vi "(SubVI)Waveform Editor_Export Manager.vi"(7 "Enable Memory":bool, 8 "error in (no error)":errorcluster caption="에러 입력(에러 없음)", 10 "Sampling Rate":u32 caption="Sampling Rate :", 11 "WF List":T1[](array[typedef])) -> (0 "error out":errorcluster caption="에러 출력")   [LabVIEW 2020]
uses:
  Controls/(Ctrl)Waveform Editor_WF List.ctl
  Libraries/Waveform Obj Class/Waveform Obj/Waveform Obj.lvclass
  <vilib>/Utility/miscctls.llb/LVPointTypeDef.ctl
  Control Data/Controls/(Ctrl)Control Data_Save or Load Control Data_Function.ctl
  <vilib>/Utility/miscctls.llb/LVStringsAndValuesArrayTypeDef_I32.ctl
  Libraries/Haptic IC Class/Haptic IC/Haptic IC.lvclass/Haptic IC.ctl
  Variables/(Var)System Variables.vi
  Libraries/Haptic IC Class/Haptic IC/Haptic IC.lvclass
panel:
  in  "Export":bool
  in  "File Format":enum32{"TXT", "WAV"}(tab)
  out "Text_Sampling Rate":u32 caption="Sampling Rate" format="%#pHz"
  in  "TXT_EOL+Delimiter":bool=TRUE
  in  "TXT_Number per Line":i32=1 caption="Number per Line" min=1 max=100
  in  "TXT_End of LIne":enum16{"EOL (\\r\\n)", "LF (\\n)"}(ring) caption="End of Line"
  in  "TXT_Delimiter":string(combo)="\r\n" caption="Delimiter"
  in  "TXT_Prefix":bool=TRUE
  in  "TXT_Waveform No.":i32(ring) caption="Waveform No."
  in  "TXT_Radix":enum16{"BIN", "DEC", "HEX"}(ring)=enum."HEX" caption="Radix"
  out "TXT_Preview":string caption="Preview"
  in  "WAV_Preview Data Type":enum16{"±1", "8bit"}(ring) caption="Preview"
  in  "WAV_Waveform No.":i32(ring) caption="Waveform No."
  out "WAV_Sampling Rate":u32 caption="Sampling Rate" format="%#pHz"
  out "WAV_Bits Per Sample":i32(ring)=8 caption="Bits / Sample" items=["8"=8, "16"=16, "24"=24, "32"=32]
  out "WAV_Preview":waveform(dbl)(graph) caption="Preview"
  # "Export Manager"
  # "Sound Format"
  # "Data Format"
  # "Preview"
  # "Data"
  # "Data Format"
  # "Data"
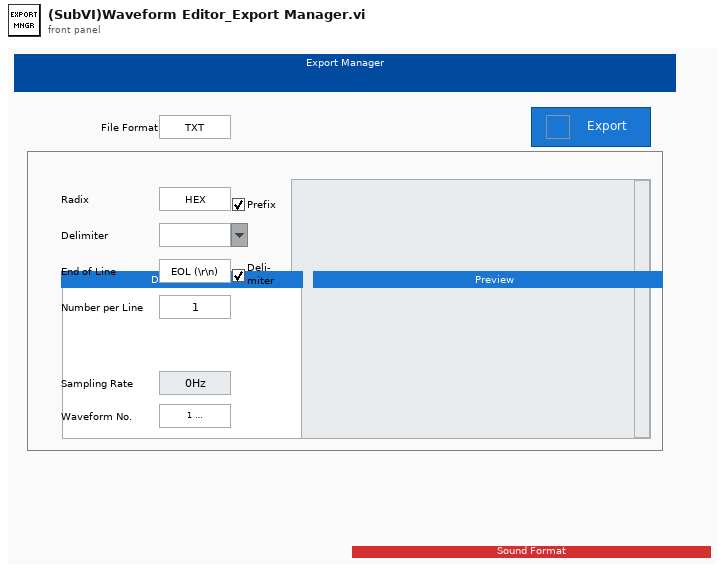
[diagram p1: front panel]
types:
  T1 = typedef "(Ctrl)Waveform Editor_WF List.ctl" = cluster{"Name":string, "WF Seq":refnum<class "Waveform Obj.lvclass">[]}
  T2 = typedef "LVPointTypeDef.ctl" = cluster{"Horizontal":i16, "Vertical":i16}
  T3 = typedef "(Ctrl)Control Data_Save or Load Control Data_Function.ctl" = enum16{"Save", "Load"}
  T4 = typedef "LVStringsAndValuesArrayTypeDef_I32.ctl" = cluster{"String":string, "Value":i32}[]
  T5 = typedef "Haptic IC.lvclass/(Ctrl)IC Type.ctl" = enum8{"DW7800", "DW7802", "DW7912", "DW7914"}
  T6 = enum8{"Enabled", "Disabled", "Disabled and Grayed Out"}
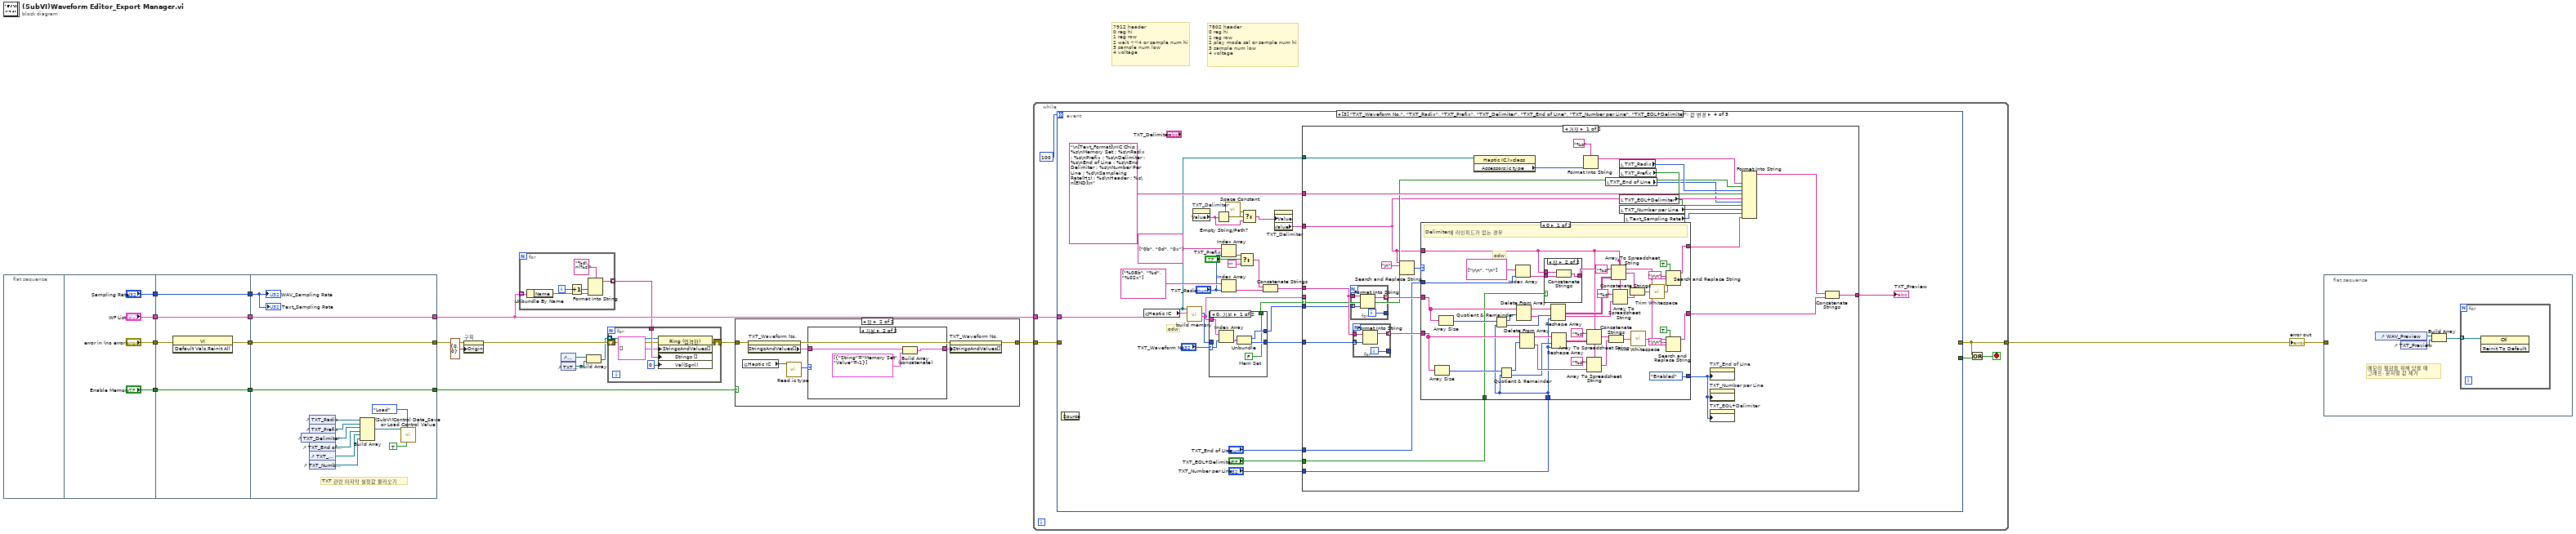
[diagram p0: block diagram]
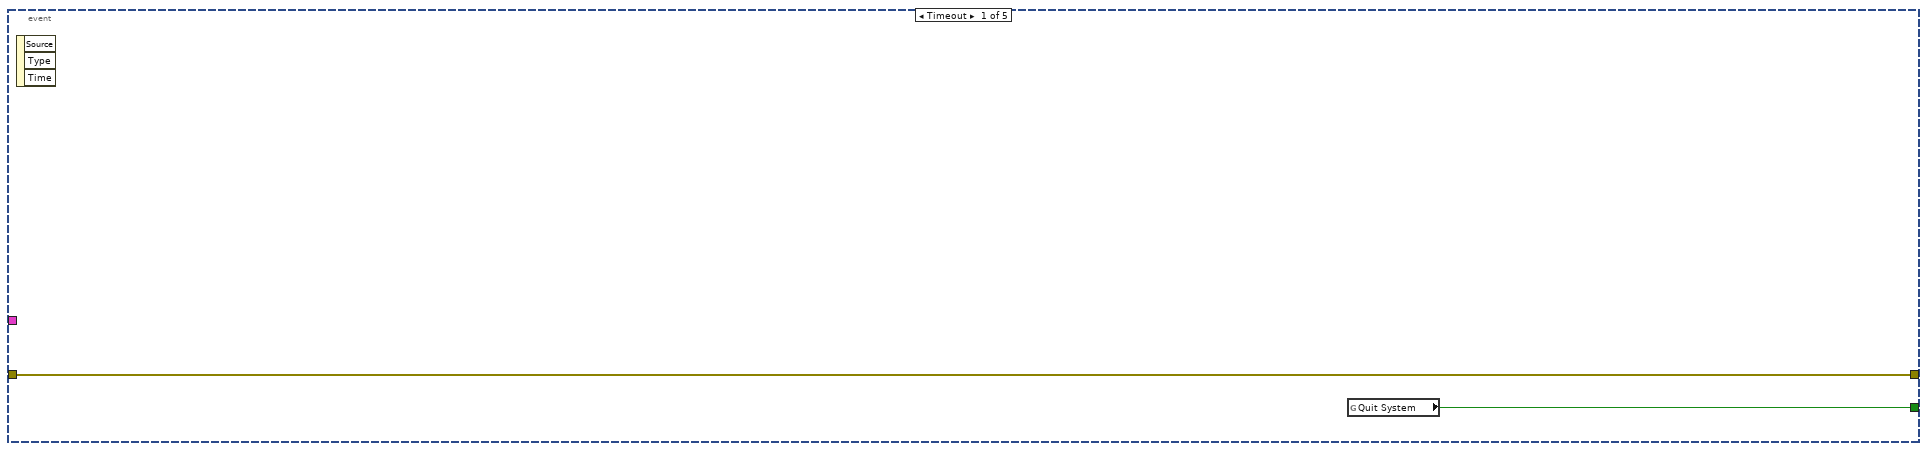
[diagram p4: hidden frame]
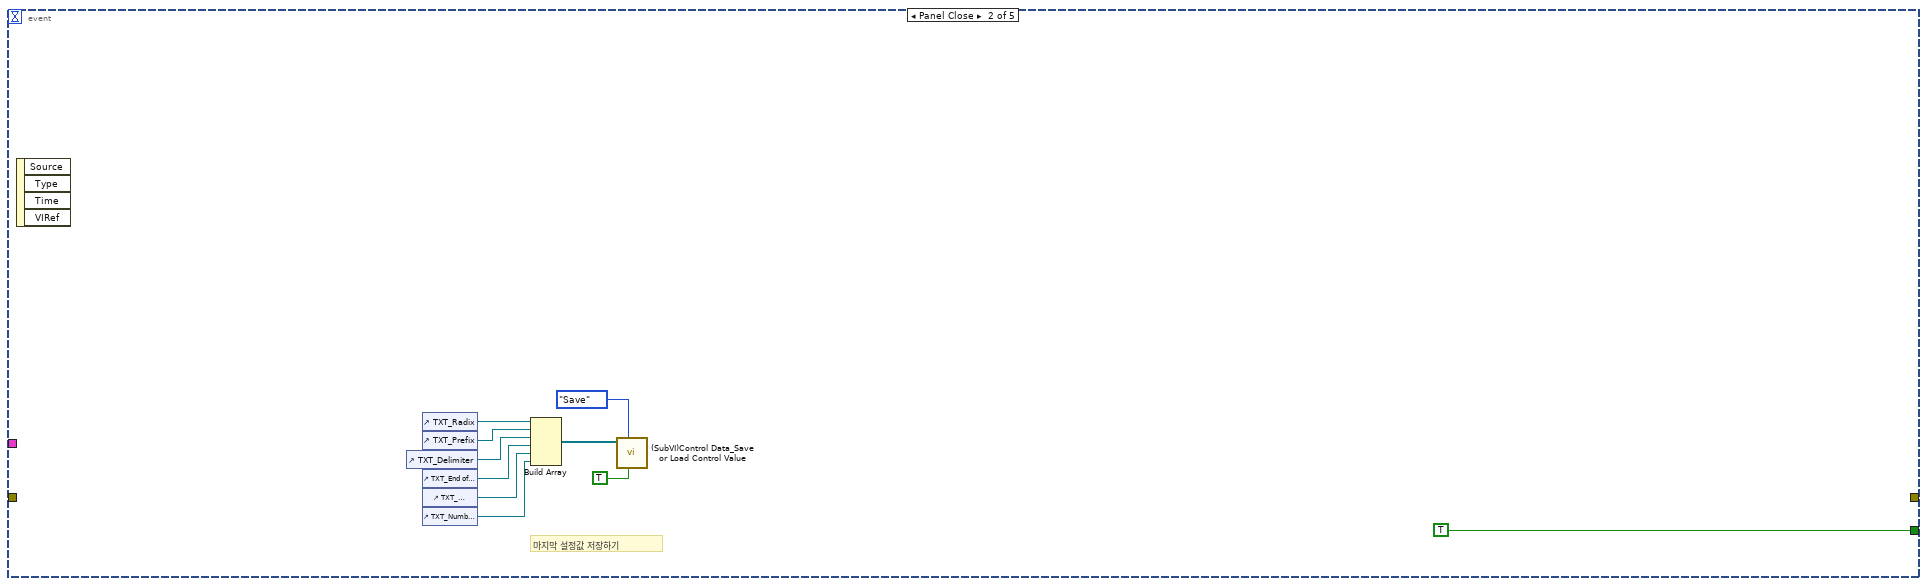
[diagram p5: hidden frame]
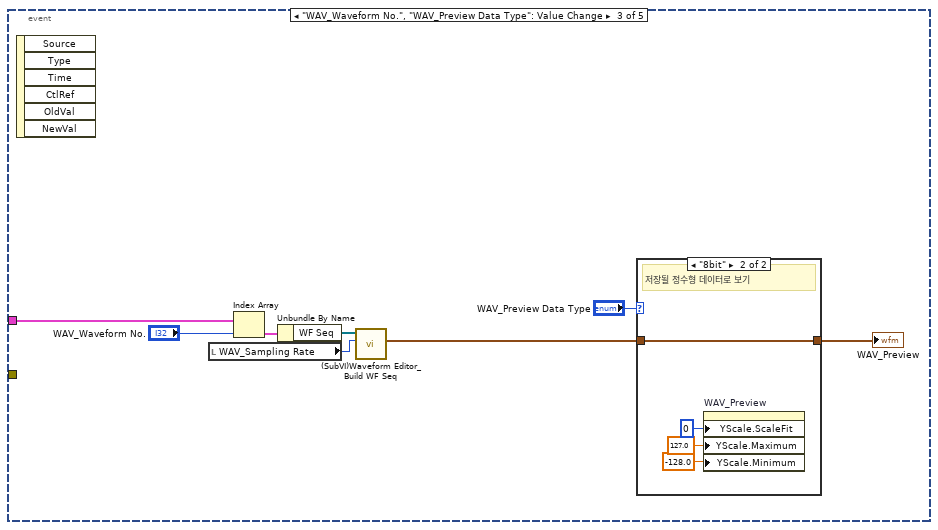
[diagram p6: hidden frame]
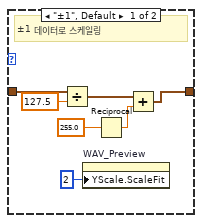
[diagram p7: hidden frame]
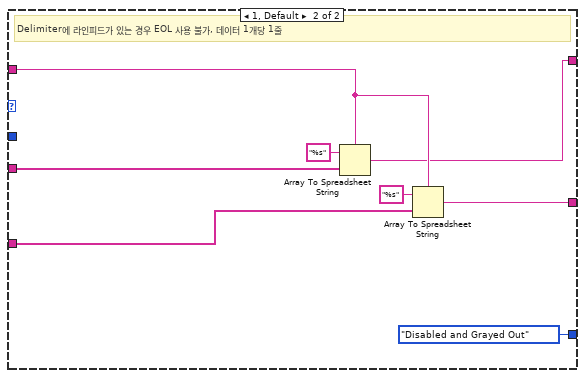
[diagram p9: hidden frame]
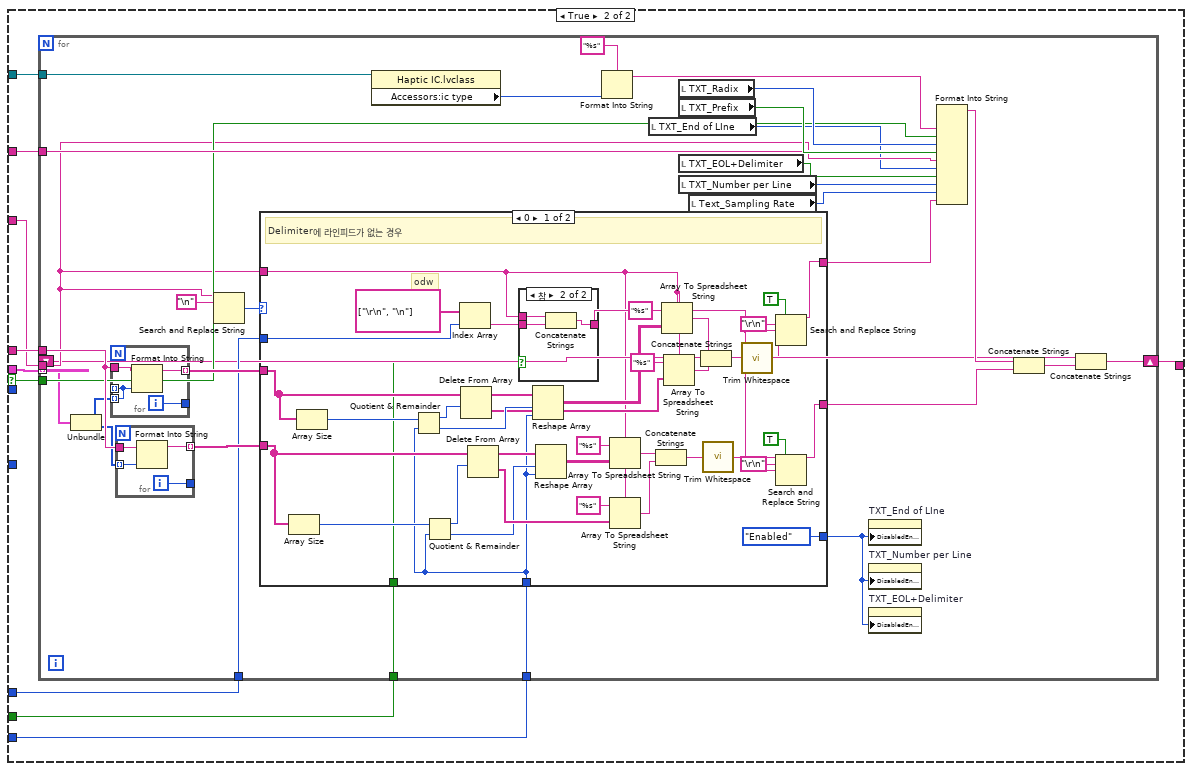
[diagram p10: hidden frame]
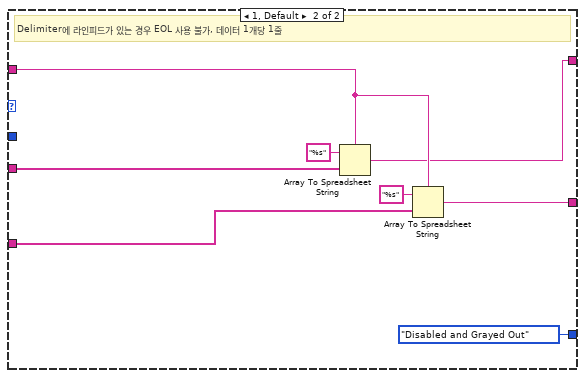
[diagram p12: hidden frame]
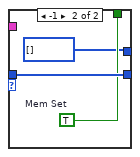
[diagram p13: hidden frame]
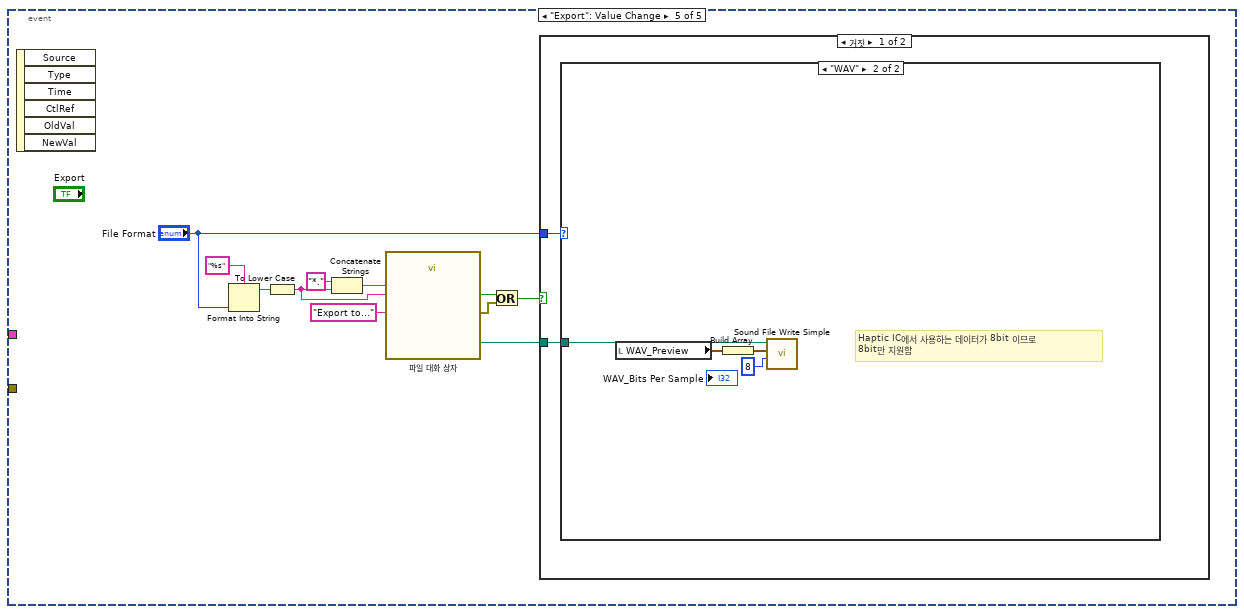
[diagram p14: hidden frame]
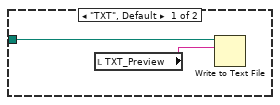
[diagram p15: hidden frame]
diagram:
  # "7802 header\n0 reg hi\n1 reg row\n2 play mode cal or sample num hi\n3 sample num low\n4 voltage"
  # "7912 header\n0 reg hi\n1 reg row\n2 wait <<4 or sample num hi\n3 sample num low\n4 voltage"
  n1 = flat-sequence {
    tunnel: ["error in (no error)"] -> w16
    tunnel: ["WF List"] -> w15
    tunnel: ["Sampling Rate"] -> w10
    tunnel: ["Enable Memory"] -> w1
    tunnel: w16 -> [w28]
    tunnel: w15 -> [w29]
    tunnel: [w29] -> w13
    tunnel: [w27] -> w12
    tunnel: [w26] -> w11
    tunnel: w10 -> [w26]
    tunnel: [w25] -> w2
    tunnel: w1 -> [w25]
    tunnel: [w41] -> w14
    tunnel: [w42] -> w19
    tunnel: w13 -> [w42]
    tunnel: w12 -> [w41]
    tunnel: w11 -> [w30]
    tunnel: [w31] -> w3
    tunnel: w2 -> [w31]
    frame #0 {
    }
    frame #1 {
    }
    frame #2 {
      n2 = invoke class="VI" method="Default Vals.Reinit All"(error in=w28) -> (error out=w27:errorcluster)  [unwired: 2 in, 2 out]
    }
    frame #3 {
      # "TXT 관련 마지막 설정값 불러오기"
      n3 = control-ref of="TXT_Delimiter"() -> (w37:refnum<vi>)
      n4 = control-ref of="TXT_Radix"() -> (w35:refnum<vi>)
      n5 = control-ref of="TXT_Prefix"() -> (w36:refnum<vi>)
      n6 = control-ref of="TXT_End of LIne"() -> (w38:refnum<vi>)
      n7 = control-ref of="TXT_EOL+Delimiter"() -> (w39:refnum<vi>)
      n8 = control-ref of="TXT_Number per Line"() -> (w40:refnum<vi>)
      n9 = Build Array(w35, w36, w37, w38, w39, w40) -> (w33:refnum<vi>[])
      n10 = call "(SubVI)Control Data_Save or Load Control Value.vi"("Common? (f)"=TRUE, "Function"=(Ctrl)Control_Data_Save_or_Load_Control_Data_Function."Load", "Control Ref"=w33) -> ()  [unwired: 8 in, 1 out]
      "WAV_Sampling Rate" <- w30
      "Text_Sampling Rate" <- w30
    }
  }
  n11 = property on="구획" class="Pane"(error in=w14, "Origin"=T2 {"Horizontal"=0, "Vertical"=0} ("원점")) -> (error out=w17:errorcluster)  [unwired: 1 in, 1 out]
  n12 = for {
    tunnel: w19 -> [w48] mode=indexing
    tunnel: [w44] -> w18 mode=indexing
    i -> [w46]
    n13 = Unbundle By Name(w48) -> ("Name"=w47:string)
    n14 = Increment(x=w46) -> (x+1=w43:i32)
    n15 = Format Into String(format string="%d\n(%s)" ("포맷 문자열"), w43, w47) -> (resulting string=w44:string)  [unwired: 2 in, 1 out]
  }
  n16 = control-ref of="WAV_Waveform No."() -> (w9:refnum<vi>)
  n17 = control-ref of="TXT_Waveform No."() -> (w8:refnum<vi>)
  n18 = Build Array(w9, w8) -> (w7:refnum<vi>[])
  n19 = for {
    tunnel: w18 -> [w54]
    tunnel: w7 -> [w50] mode=indexing
    shift-right: [w52] -> w5
    shift-left: w17 -> [w53]
    n20 = property on="프로퍼티 노드" class="Ring (엄격한)"(reference=w50, error in=w53, "StringsAndValues[]"=T4 [] ("문자열과 값[]"), "Strings []"=w54, "Val(Sgnl)"=0 ("값(신호)")) -> (error out=w52:errorcluster)  [unwired: 1 out]
  }
  n21 = case shown="참" w3 {
    tunnel: w5 -> [w55 w62]
    tunnel: [w55 w60] -> w4
    frame False {
    }
    frame True {
      n22 = global read "(Var)System Variables.vi" "Haptic IC"() -> (w57:refnum<class "Haptic IC.lvclass">)
      n23 = property on="TXT_Waveform No." class="Ring (엄격한)"(error in=w62) -> (error out=w61:errorcluster, "StringsAndValues[]"=w59:T4)  [unwired: 1 in, 1 out]
      n24 = call "Read ic type.vi"("Haptic IC 입력"=w57) -> ("ic type"=w56:T5)  [unwired: 8 in, 2 out]
      n25 = case shown="기본" w56 {
        tunnel: w59 -> [w63 w66]
        tunnel: [w63 w64] -> w58
        frame "DW7800" {
          # "Memory를 사용하지 않는 IC의 경우 (DW7800)\nMemory Set 없이 개별 Waveform 데이터만 사용"
        }
        frame Default {
          n26 = Build Array (concatenate)(w66, T4 [{"String"="Memory Set", "Value"=-1}] ("배열")) -> (w64:T4)
        }
      }
      n27 = property on="TXT_Waveform No." class="Ring (엄격한)"(error in=w61, "StringsAndValues[]"=w58) -> (error out=w60:errorcluster)  [unwired: 1 in, 1 out]
    }
  }
  n28 = while {
    tunnel: w4 -> [w71]
    tunnel: [w70] -> w6
    tunnel: w19 -> [w67]
    stop <- w69 stop-if-true
    n29 = event shown="[3] \"TXT_Waveform No.\", \"TXT_Radix\", \"TXT_Prefix\", \"TXT_Delimiter\", \"TXT_End of LIne\", \"TXT_Number per Line\", \"TXT_EOL+Delimiter\": 값 변경" {
      selector: _ -> [_ _ _ _ _]
      dyn-events: _ -> [_ _ _ _ _]
      timeout: 100 -> [_ _ _ _ _]
      tunnel: [w74 _ _ _ _] -> w70
      tunnel: w71 -> [w74 _ _ _ _]
      tunnel: [w73 TRUE _ _ _] -> w68
      tunnel: w67 -> [_ _ w92 w115 _]
      event Timeout {
        n30 = event-data() -> ()  [unwired: 1 in, 3 out]
        n31 = global read "(Var)System Variables.vi" "Quit System"() -> (w73:bool)
      }
      event Panel Close {
        # "마지막 설정값 저장하기"
        n32 = event-data() -> ()  [unwired: 1 in, 4 out]
        n33 = control-ref of="TXT_Delimiter"() -> (w78:refnum<vi>)
        n34 = control-ref of="TXT_Radix"() -> (w80:refnum<vi>)
        n35 = control-ref of="TXT_Prefix"() -> (w79:refnum<vi>)
        n36 = control-ref of="TXT_End of LIne"() -> (w77:refnum<vi>)
        n37 = control-ref of="TXT_EOL+Delimiter"() -> (w76:refnum<vi>)
        n38 = control-ref of="TXT_Number per Line"() -> (w75:refnum<vi>)
        n39 = Build Array(w80, w79, w78, w77, w76, w75) -> (w82:refnum<vi>[])
        n40 = call "(SubVI)Control Data_Save or Load Control Value.vi"("Common? (f)"=TRUE, "Function"=(Ctrl)Control_Data_Save_or_Load_Control_Data_Function."Save", "Control Ref"=w82) -> ()  [unwired: 8 in, 1 out]
      }
      event "WAV_Waveform No.", "WAV_Preview Data Type": Value Change {
        n41 = event-data() -> ()  [unwired: 1 in, 6 out]
        n42 = local read "WAV_Sampling Rate"() -> (w87:u32)
        n43 = Index Array(array=w92, index="WAV_Waveform No.") -> (element=w90:T1)
        n44 = Unbundle By Name(w90) -> ("WF Seq"=w89:refnum<class "Waveform Obj.lvclass">[])
        n45 = call "(SubVI)Waveform Editor_Build WF Seq.vi"("Sampling Rate"=w87, "WF Seq"=w89) -> ("waveform out"=w86:waveform(i8))  [unwired: 4 in, 5 out]
        n46 = case shown="\"8bit\"" "WAV_Preview Data Type" {
          tunnel: w86 -> [w98 w103]
          tunnel: [w94 w103] -> w88
          frame "±1", Default {
            # "±1 데이터로 스케일링"
            n47 = Divide(x=w98, y=127.5) -> (x/y=w97:waveform(dbl))
            n48 = property on="WAV_Preview" class="WFGraph (엄격한)"("YScale.ScaleFit"=u8 2 ("Y 스케일.스케일 맞춤")) -> ()  [unwired: 2 in, 2 out]
            n49 = Reciprocal(x=255.0) -> (1/x=w95:dbl)
            n50 = Add(x=w97, y=w95) -> (x+y=w94:waveform(dbl))
          }
          frame "8bit" {
            # "저장될 정수형 데이터로 보기"
            n51 = property on="WAV_Preview" class="WFGraph (엄격한)"("YScale.ScaleFit"=u8 0 ("Y 스케일.스케일 맞춤"), "YScale.Maximum"=127.0 ("Y 스케일.범위:최대값"), "YScale.Minimum"=-128.0 ("Y 스케일.범위:최소값")) -> ()  [unwired: 2 in, 2 out]
          }
        }
        "WAV_Preview" <- w88
      }
      event "TXT_Waveform No.", "TXT_Radix", "TXT_Prefix", "TXT_Delimiter", "TXT_End of LIne", "TXT_Number per Line", "TXT_EOL+Delimiter": Value Change {
        # "odw"
        n52 = event-data() -> ()  [unwired: 1 in, 1 out]
        n53 = global read "(Var)System Variables.vi" "Haptic IC"() -> (w114:refnum<class "Haptic IC.lvclass">)
        n54 = call-dynamic "build memory.vi"("WF List"=w115, "Haptic IC 입력"=w114) -> ("memory data by wf"=w104:cluster{"Header":u8[], "Data":u8[]}[], "full memory data"=w108:u8[])  [unwired: 6 in, 2 out]
        n55 = property on="TXT_Delimiter" class="CmbBox"() -> ("Value"=w111:string)  [unwired: 2 in, 2 out]
        n56 = case shown="0, 기본" "TXT_Waveform No." {
          selector: "TXT_Waveform No." -> [w324 _]
          tunnel: [w322 w328] -> w129
          tunnel: w108 -> [_ w328]
          tunnel: w104 -> [w325 _]
          tunnel: [w321 u8[] [] ("Header")] -> w118
          tunnel: [w320 w327] -> w116
          frame 0, Default {
            w320 = FALSE  # Mem Set
            n57 = Index Array(array=w325, index=w324) -> (element=w323:cluster{"Header":u8[], "Data":u8[]})
            n58 = Unbundle(w323) -> ("Header"=w321:u8[], "Data"=w322:u8[])
          }
          frame -1 {
            w327 = TRUE  # Mem Set
          }
        }
        n59 = Empty String/Path?(string/path=w111) -> (empty?=w113:bool)
        n60 = Index Array(array=string[] ["0b", "0d", "0x"], index="TXT_Radix") -> (element=w126:string)
        n61 = Index Array(array=string[] ["%08b", "%d", "%02x"], index="TXT_Radix") -> (element=w124:string)
        n62 = call <vilib>:"Space Constant.vi"() -> ("String"=w112:string)
        n63 = Select(t=w126, s="TXT_Prefix", f="") -> (s? t:f=w123:string)
        n64 = Select(t=w112, s=w113, f=w111) -> (s? t:f=w110:string)
        n65 = Concatenate Strings(w123, w124) -> (w119:string)
        n66 = property on="TXT_Delimiter" class="CmbBox"("Value"=w110) -> ("Value"=w109:string)  [unwired: 2 in, 2 out]
        n67 = case shown="거짓" w116 {
          selector: w116 -> [w143 w226]
          tunnel: w129 -> [w157 _]
          tunnel: [w149 w219] -> w120
          tunnel: w119 -> [w147 w228]
          tunnel: w118 -> [w146 _]
          tunnel: "\n[Text_Format]\nIC Chip : %s\nMemory Set : %s\nRadix : %s\nPrefix : %s\nDelimiter : %s\nEnd of Line : %s\nEnd Delimiter : %s\nNumber Per Line : %d\nSampleing Rate(Hz) : %d\nHeader : %s\n[END]\n" ("포맷 문자열") -> [w144 w227]
          tunnel: w114 -> [w142 w225]
          tunnel: w109 -> [w136 w224]
          tunnel: "TXT_Number per Line" -> [w133 w223]
          tunnel: "TXT_EOL+Delimiter" -> [w132 w222]
          tunnel: "TXT_End of LIne" -> [w131 w221]
          tunnel: w104 -> [_ w220]
          frame False {
            n68 = for {
              tunnel: w147 -> [w162]
              tunnel: [w161] -> w145 mode=indexing
              tunnel: [w160] -> _
              tunnel: w146 -> [w159] mode=indexing
              i -> [w160]
              n69 = Format Into String(format string=w162, w159) -> (resulting string=w161:string)  [unwired: 2 in, 1 out]
            }
            n70 = for {
              tunnel: w157 -> [w166] mode=indexing
              tunnel: w147 -> [w165]
              tunnel: [w164] -> w156 mode=indexing
              tunnel: [w163] -> _
              i -> [w163]
              n71 = Format Into String(format string=w165, w166) -> (resulting string=w164:string)  [unwired: 2 in, 1 out]
            }
            n72 = Search and Replace String(input string=w136, search string="\n") -> (number of replacements=w154:i32)  [unwired: 6 in, 3 out]
            n73 = case shown="0" w154 {
              tunnel: w156 -> [w206 w217]
              tunnel: w136 -> [w175 w212]
              tunnel: [w201 w216] -> w134
              tunnel: [T6."Enabled" ("비활성화") T6."Disabled and Grayed Out" ("비활성화")] -> w155
              tunnel: w145 -> [w181 w213]
              tunnel: [w182 w211] -> w138
              tunnel: w133 -> [w169 _]
              tunnel: w132 -> [w168 _]
              tunnel: w131 -> [w167 _]
              frame 0 {
                # "odw"
                # "Delimiter에 라인피드가 없는 경우"
                n74 = Array Size(array=w206) -> (size(s)=w205:i32)
                n75 = Array Size(array=w181) -> (size(s)=w180:i32)
                n76 = Quotient & Remainder(x=w180, y=w169) -> (x-y*floor(x/y)=w179:i32, floor(x/y)=w178:i32)
                n77 = Quotient & Remainder(x=w205, y=w169) -> (x-y*floor(x/y)=w189:i32, floor(x/y)=w187:i32)
                n78 = Index Array(array=string[] ["\r\n", "\n"], index=w167) -> (element=w170:string)
                n79 = Delete From Array(array=w181, length=w179) -> (deleted portion=w176:string[], array with subset deleted=w188:string[])  [unwired: 1 in]
                n80 = Delete From Array(array=w206, length=w189) -> (deleted portion=w194:string[], array with subset deleted=w196:string[])  [unwired: 1 in]
                n81 = case shown="참" w168 {
                  tunnel: w170 -> [w207 w210]
                  tunnel: w175 -> [_ w209]
                  tunnel: [w207 w208] -> w183
                  frame False {
                  }
                  frame True {
                    n82 = Concatenate Strings(w209, w210) -> (w208:string)
                  }
                }
                n83 = Reshape Array(w188, w178, w169) -> (w186:string[][])
                n84 = Reshape Array(w196, w187, w169) -> (w203:string[][])
                n85 = Array To Spreadsheet String(delimiter (Tab)=w175, array=w203, 3:"%s" ("포맷 문자열")) -> (spreadsheet string=w202:string)
                n86 = Array To Spreadsheet String(delimiter (Tab)=w175, array=w194, 3:"%s" ("포맷 문자열")) -> (spreadsheet string=w192:string)
                n87 = Concatenate Strings(w202, w192) -> (w193:string)
                n88 = Array To Spreadsheet String(delimiter (Tab)=w175, array=w186, 3:"%s" ("포맷 문자열")) -> (spreadsheet string=w174:string)
                n89 = Array To Spreadsheet String(delimiter (Tab)=w175, array=w176, 3:"%s" ("포맷 문자열")) -> (spreadsheet string=w173:string)
                n90 = Concatenate Strings(w174, w173) -> (w172:string)
                n91 = call <vilib>:"Trim Whitespace.vi"("string"=w193) -> ("trimmed string"=w191:string)  [unwired: 1 in]
                n92 = call <vilib>:"Trim Whitespace.vi"("string"=w172) -> ("trimmed string"=w171:string)  [unwired: 1 in]
                n93 = Search and Replace String(replace all?=TRUE ("모두 대체? (거짓)"), input string=w171, search string="\r\n" ("검색 문자열"), replace string=w183) -> (result string=w182:string)  [unwired: 4 in, 3 out]
                n94 = Search and Replace String(replace all?=TRUE ("모두 대체? (거짓)"), input string=w191, search string="\r\n" ("검색 문자열"), replace string=w183) -> (result string=w201:string)  [unwired: 4 in, 3 out]
              }
              frame 1, Default {
                # "Delimiter에 라인피드가 있는 경우 EOL 사용 불가, 데이터 1개당 1줄"
                n95 = Array To Spreadsheet String(delimiter (Tab)=w212, array=w213, 3:"%s" ("포맷 문자열")) -> (spreadsheet string=w211:string)
                n96 = Array To Spreadsheet String(delimiter (Tab)=w212, array=w217, 3:"%s" ("포맷 문자열")) -> (spreadsheet string=w216:string)
              }
            }
            n97 = property class="Haptic IC.lvclass"(reference=w142) -> ("Accessors:ic type"=w141:T5)  [unwired: 1 in, 2 out]
            n98 = Format Into String(format string="%s" ("포맷 문자열"), w141) -> (resulting string=w139:string)  [unwired: 2 in, 1 out]
            n99 = local read "TXT_End of LIne"() -> (w135:enum16{"EOL (\\r\\n)", "LF (\\n)"})
            n100 = local read "TXT_Radix"() -> (w148:enum16{"BIN", "DEC", "HEX"})
            n101 = local read "TXT_Prefix"() -> (w153:bool)
            n102 = local read "TXT_EOL+Delimiter"() -> (w152:bool)
            n103 = local read "TXT_Number per Line"() -> (w151:i32)
            n104 = local read "Text_Sampling Rate"() -> (w137:u32)
            n105 = property on="TXT_End of LIne" class="Enum (엄격한)"("DisabledEnum"=w155) -> ()  [unwired: 2 in, 2 out]
            n106 = property on="TXT_Number per Line" class="DigNum (엄격한)"("DisabledEnum"=w155) -> ()  [unwired: 2 in, 2 out]
            n107 = property on="TXT_EOL+Delimiter" class="Bool (엄격한)"("DisabledEnum"=w155) -> ()  [unwired: 2 in, 2 out]
            n108 = Format Into String(format string=w144, w139, w143, w148, w153, w136, w135, w152, w151, w137, w138) -> (resulting string=w150:string)  [unwired: 2 in, 1 out]
            n109 = Concatenate Strings(w150, w134) -> (w149:string)
          }
          frame True {
            n110 = for {
              tunnel: w228 -> [w250]
              tunnel: w227 -> [w248]
              tunnel: w226 -> [w247]
              tunnel: w225 -> [w246]
              tunnel: w223 -> [w237]
              tunnel: w222 -> [w236]
              tunnel: w221 -> [w235]
              tunnel: w220 -> [w234] mode=indexing
              tunnel: w224 -> [w240]
              shift-right: [w230] -> w219
              shift-left: _ -> [w229]
              n111 = Unbundle(w234) -> ("Header"=w233:u8[], "Data"=w232:u8[])
              n112 = for {
                tunnel: w250 -> [w263]
                tunnel: [w262] -> w249 mode=indexing
                tunnel: [w261] -> _
                tunnel: [w260] -> _ mode=indexing
                tunnel: w233 -> [w260] mode=indexing
                i -> [w261]
                n113 = Format Into String(format string=w263, w260) -> (resulting string=w262:string)  [unwired: 2 in, 1 out]
              }
              n114 = for {
                tunnel: w232 -> [w267] mode=indexing
                tunnel: w250 -> [w266]
                tunnel: [w265] -> w258 mode=indexing
                tunnel: [w264] -> _
                i -> [w264]
                n115 = Format Into String(format string=w266, w267) -> (resulting string=w265:string)  [unwired: 2 in, 1 out]
              }
              n116 = Search and Replace String(input string=w240, search string="\n") -> (number of replacements=w256:i32)  [unwired: 6 in, 3 out]
              n117 = case shown="0" w256 {
                tunnel: w258 -> [w307 w318]
                tunnel: w240 -> [w276 w313]
                tunnel: [w302 w317] -> w238
                tunnel: [T6."Enabled" ("비활성화") T6."Disabled and Grayed Out" ("비활성화")] -> w257
                tunnel: w249 -> [w282 w314]
                tunnel: [w283 w312] -> w242
                tunnel: w237 -> [w270 _]
                tunnel: w236 -> [w269 _]
                tunnel: w235 -> [w268 _]
                frame 0 {
                  # "odw"
                  # "Delimiter에 라인피드가 없는 경우"
                  n118 = Array Size(array=w307) -> (size(s)=w306:i32)
                  n119 = Array Size(array=w282) -> (size(s)=w281:i32)
                  n120 = Quotient & Remainder(x=w281, y=w270) -> (x-y*floor(x/y)=w280:i32, floor(x/y)=w279:i32)
                  n121 = Quotient & Remainder(x=w306, y=w270) -> (x-y*floor(x/y)=w290:i32, floor(x/y)=w288:i32)
                  n122 = Index Array(array=string[] ["\r\n", "\n"], index=w268) -> (element=w271:string)
                  n123 = Delete From Array(array=w282, length=w280) -> (deleted portion=w277:string[], array with subset deleted=w289:string[])  [unwired: 1 in]
                  n124 = Delete From Array(array=w307, length=w290) -> (deleted portion=w295:string[], array with subset deleted=w297:string[])  [unwired: 1 in]
                  n125 = case shown="참" w269 {
                    tunnel: w271 -> [w308 w311]
                    tunnel: w276 -> [_ w310]
                    tunnel: [w308 w309] -> w284
                    frame False {
                    }
                    frame True {
                      n126 = Concatenate Strings(w310, w311) -> (w309:string)
                    }
                  }
                  n127 = Reshape Array(w289, w279, w270) -> (w287:string[][])
                  n128 = Reshape Array(w297, w288, w270) -> (w304:string[][])
                  n129 = Array To Spreadsheet String(delimiter (Tab)=w276, array=w304, 3:"%s" ("포맷 문자열")) -> (spreadsheet string=w303:string)
                  n130 = Array To Spreadsheet String(delimiter (Tab)=w276, array=w295, 3:"%s" ("포맷 문자열")) -> (spreadsheet string=w293:string)
                  n131 = Concatenate Strings(w303, w293) -> (w294:string)
                  n132 = Array To Spreadsheet String(delimiter (Tab)=w276, array=w287, 3:"%s" ("포맷 문자열")) -> (spreadsheet string=w275:string)
                  n133 = Array To Spreadsheet String(delimiter (Tab)=w276, array=w277, 3:"%s" ("포맷 문자열")) -> (spreadsheet string=w274:string)
                  n134 = Concatenate Strings(w275, w274) -> (w273:string)
                  n135 = call <vilib>:"Trim Whitespace.vi"("string"=w294) -> ("trimmed string"=w292:string)  [unwired: 1 in]
                  n136 = call <vilib>:"Trim Whitespace.vi"("string"=w273) -> ("trimmed string"=w272:string)  [unwired: 1 in]
                  n137 = Search and Replace String(replace all?=TRUE ("모두 대체? (거짓)"), input string=w272, search string="\r\n" ("검색 문자열"), replace string=w284) -> (result string=w283:string)  [unwired: 4 in, 3 out]
                  n138 = Search and Replace String(replace all?=TRUE ("모두 대체? (거짓)"), input string=w292, search string="\r\n" ("검색 문자열"), replace string=w284) -> (result string=w302:string)  [unwired: 4 in, 3 out]
                }
                frame 1, Default {
                  # "Delimiter에 라인피드가 있는 경우 EOL 사용 불가, 데이터 1개당 1줄"
                  n139 = Array To Spreadsheet String(delimiter (Tab)=w313, array=w314, 3:"%s" ("포맷 문자열")) -> (spreadsheet string=w312:string)
                  n140 = Array To Spreadsheet String(delimiter (Tab)=w313, array=w318, 3:"%s" ("포맷 문자열")) -> (spreadsheet string=w317:string)
                }
              }
              n141 = property class="Haptic IC.lvclass"(reference=w246) -> ("Accessors:ic type"=w245:T5)  [unwired: 1 in, 2 out]
              n142 = Format Into String(format string="%s" ("포맷 문자열"), w245) -> (resulting string=w243:string)  [unwired: 2 in, 1 out]
              n143 = local read "TXT_End of LIne"() -> (w239:enum16{"EOL (\\r\\n)", "LF (\\n)"})
              n144 = local read "TXT_Radix"() -> (w251:enum16{"BIN", "DEC", "HEX"})
              n145 = local read "TXT_Prefix"() -> (w255:bool)
              n146 = local read "TXT_EOL+Delimiter"() -> (w254:bool)
              n147 = local read "TXT_Number per Line"() -> (w253:i32)
              n148 = local read "Text_Sampling Rate"() -> (w241:u32)
              n149 = property on="TXT_End of LIne" class="Enum (엄격한)"("DisabledEnum"=w257) -> ()  [unwired: 2 in, 2 out]
              n150 = property on="TXT_Number per Line" class="DigNum (엄격한)"("DisabledEnum"=w257) -> ()  [unwired: 2 in, 2 out]
              n151 = property on="TXT_EOL+Delimiter" class="Bool (엄격한)"("DisabledEnum"=w257) -> ()  [unwired: 2 in, 2 out]
              n152 = Format Into String(format string=w248, w243, w247, w251, w255, w240, w239, w254, w253, w241, w242) -> (resulting string=w252:string)  [unwired: 2 in, 1 out]
              n153 = Concatenate Strings(w252, w238) -> (w231:string)
              n154 = Concatenate Strings(w229, w231) -> (w230:string)
            }
          }
        }
        "TXT_Preview" <- w120
      }
      event "Export": Value Change {
        n155 = event-data() -> ()  [unwired: 1 in, 6 out]
        n156 = Format Into String(format string="%s" ("포맷 문자열"), "File Format") -> (resulting string=w337:string)  [unwired: 2 in, 1 out]
        n157 = To Lower Case(string=w337) -> (all lower case string=w334:string)
        n158 = Concatenate Strings("*." ("문자열"), w334) -> (w335:string)
        n159 = call "파일 대화 상자"("prompt"="Export to...", "pattern (all files)"=w335, "pattern label"=w334) -> ("selected path"=w332:path, "cancelled"=w331:bool, "error out"=w330:errorcluster)  [unwired: 9 in, 1 out]
        n160 = Or(x=w331, y=w330) -> (x .or. y?=w329:bool)
        n161 = case shown="거짓" w329 {
          tunnel: "File Format" -> [w341 _]
          tunnel: w332 -> [w340 _]
          frame False {
            n162 = case shown="\"WAV\"" w341 {
              tunnel: w340 -> [w343 w347]
              frame "TXT", Default {
                n163 = local read "TXT_Preview"() -> (w342:string)
                n164 = Write to Text File(file (use dialog)=w343, text=w342) -> ()  [unwired: 2 in, 3 out]
              }
              frame "WAV" {
                # "Haptic IC에서 사용하는 데이터가 8bit 이므로\n8bit만 지원함"
                n165 = local read "WAV_Preview"() -> (w346:waveform(dbl))
                n166 = Build Array(w346) -> (w345:waveform(dbl)[])
                n167 = call <vilib>:"Sound File Write Simple.vi"("bits per sample"=8, "data"=w345, "path"=w347) -> ()  [unwired: 7 in, 2 out]
              }
            }
          }
          frame True {
          }
        }
      }
    }
    n168 = Or(x=w70, y=w68) -> (x .or. y?=w69:bool)
  }
  "error out" <- w6
  n169 = flat-sequence {
    tunnel: w6 -> [_]
    frame #0 {
      # "메모리 절감을 위해 닫을 때 \n그래프, 문자열 값 제거"
      n170 = control-ref of="WAV_Preview"() -> (w349:refnum<vi>)
      n171 = control-ref of="TXT_Preview"() -> (w350:refnum<vi>)
      n172 = Build Array(w349, w350) -> (w348:refnum<vi>[])
      n173 = for {
        tunnel: w348 -> [w351] mode=indexing
        n174 = invoke class="Ctl" method="Reinit To Default"(reference=w351) -> ()  [unwired: 2 in, 3 out]
      }
    }
  }
